vi "unset seq channel writer or reader.vi"(7 "action GUID":string, 8 "error in":errorcluster, 9 "action channel":refnum<class "TBM channel.lvclass">, 10 "seq channel":refnum<class "TBM channel.lvclass">, 11 "engine configuration in":refnum<class "base TBM sequencer configuration.lvclass">) -> (0 "error out":errorcluster, 3 "engine configuration out":refnum<class "base TBM sequencer configuration.lvclass">)   [LabVIEW 2014, in "base TBM sequencer configuration.lvclass"]
uses:
  base TBM sequencer configuration.lvclass
  <vilib>/NI/Tag Bus Module Framework/channel/TBM channel.lvclass
  <vilib>/NI/Tag Bus/tag/tag descriptor.lvclass/tag descriptor.ctl
  base TBM sequencer configuration.lvclass/base TBM sequencer configuration.ctl
  <vilib>/NI/Tag Bus Module Framework/channel/TBM channel.lvclass/TBM channel.ctl
  <vilib>/NI/Tag Bus/tag/read tag name.vi
  <vilib>/NI/Tag Bus Module Framework/channel/Read channel classification.vi
  <vilib>/NI/Configuration Framework/NISE_CEF_TreeControl.lvlib
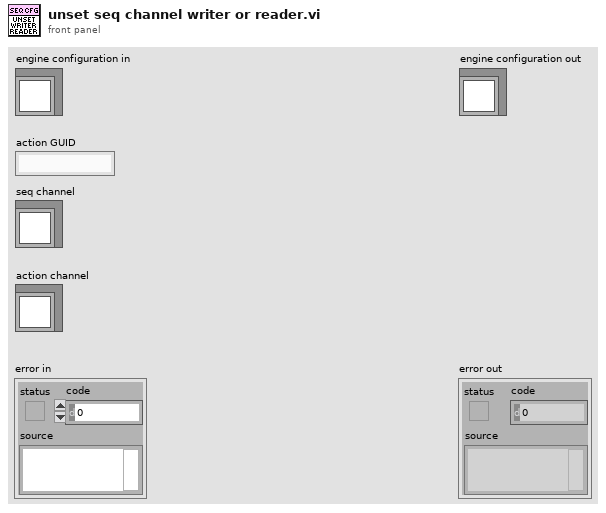
[diagram p1: front panel]
types:
  T1 = typedef "base TBM sequencer configuration.lvclass/Tag Info.ctl" = cluster{"Channel":refnum<class "TBM channel.lvclass">, "Writers":string[], "Readers":string[], "Owning ID":string}
  T2 = typedef "TBM channel.lvclass/channel classification.ctl" = enum16{"input data", "output data", "processing parameter", "processing result"}
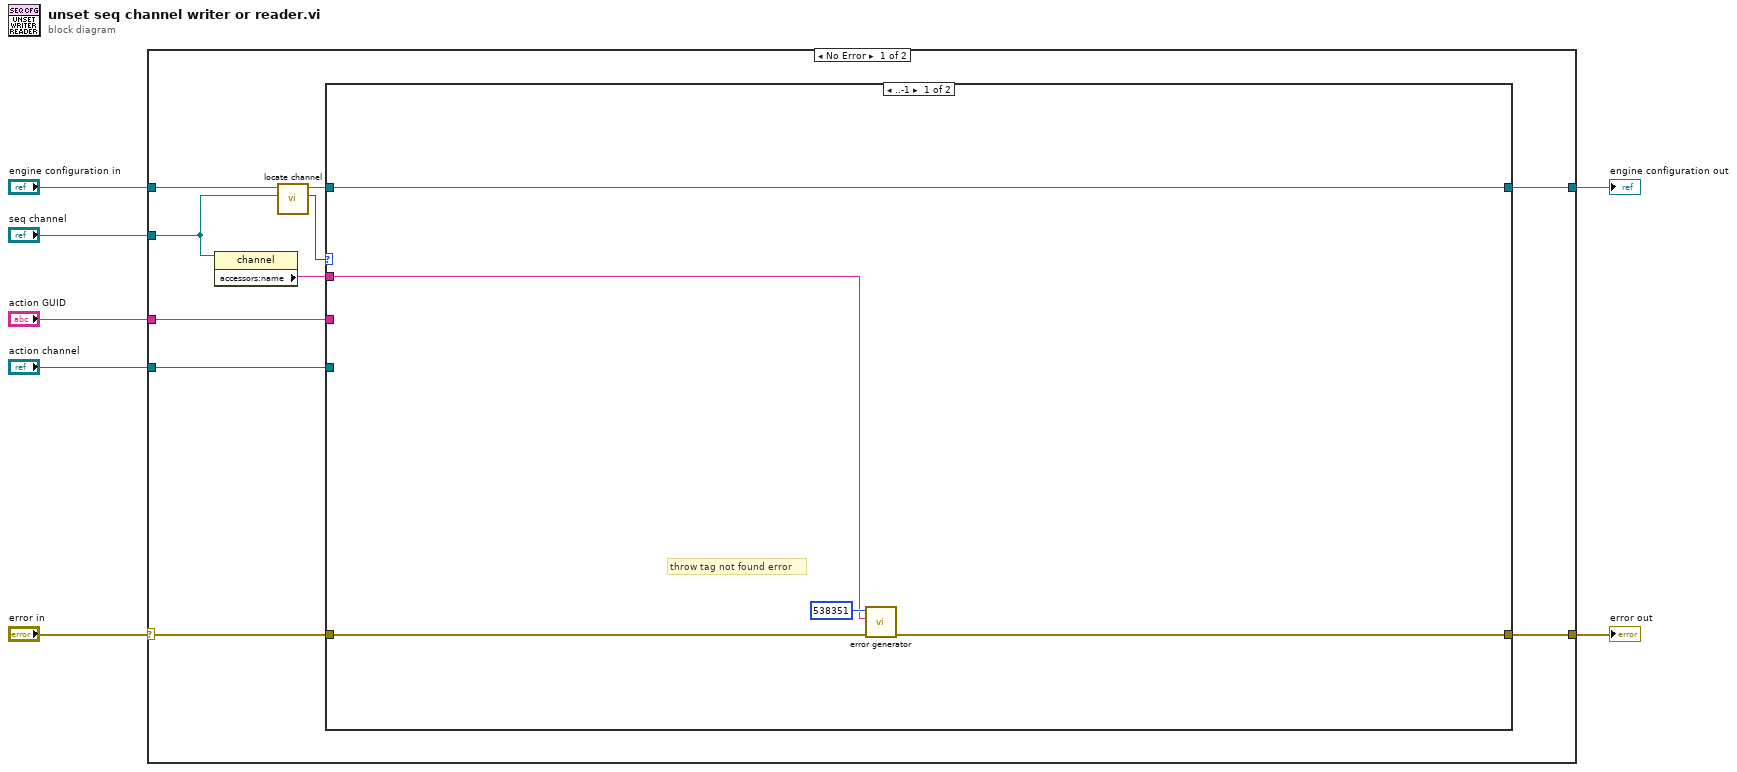
[diagram p0: block diagram]
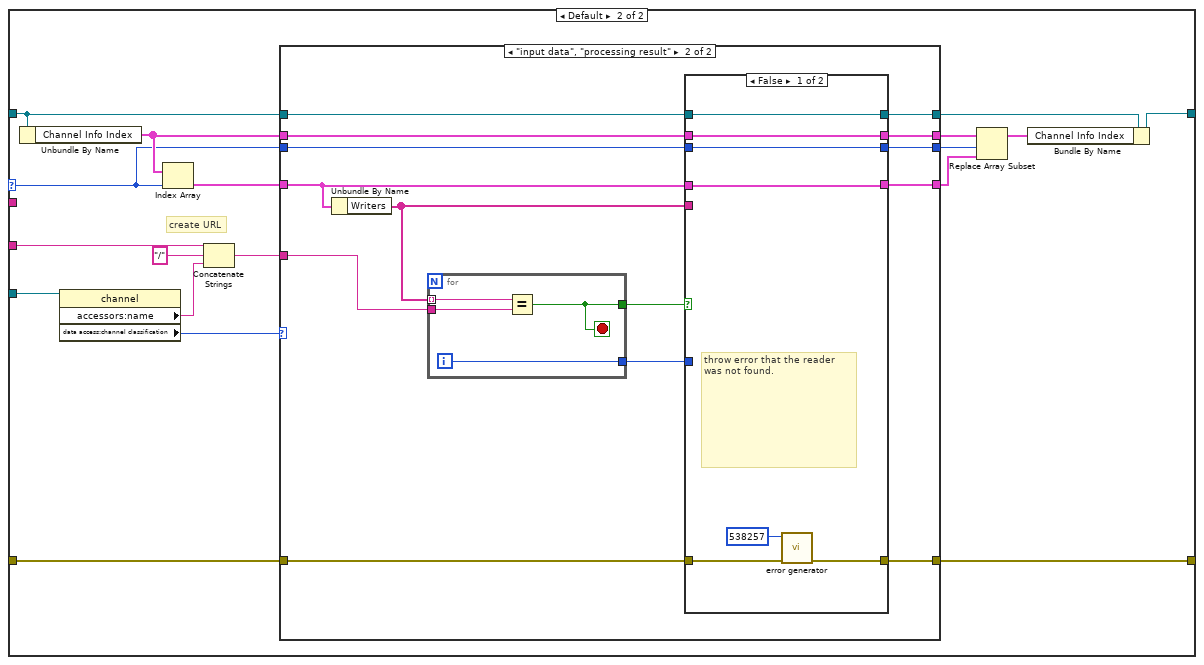
[diagram p2: hidden frame]
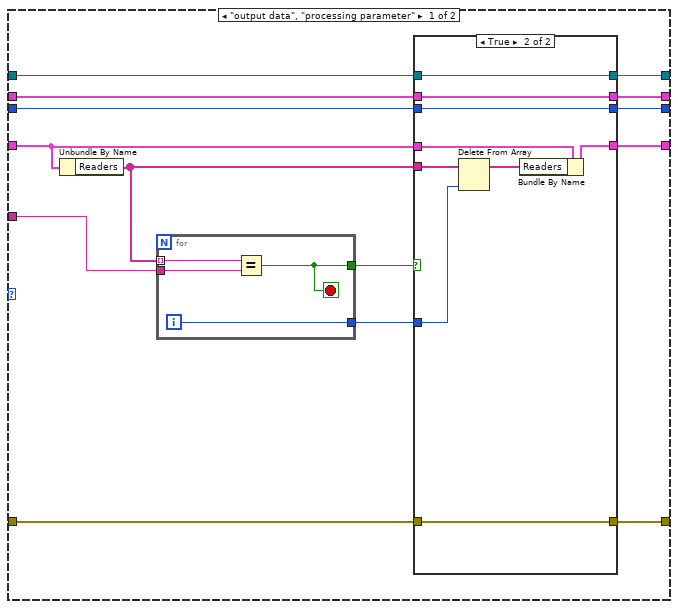
[diagram p3: hidden frame]
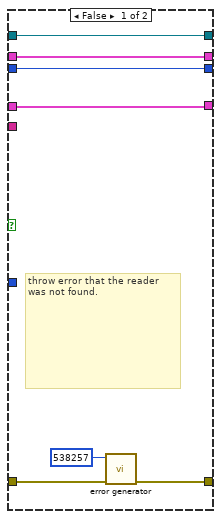
[diagram p4: hidden frame]
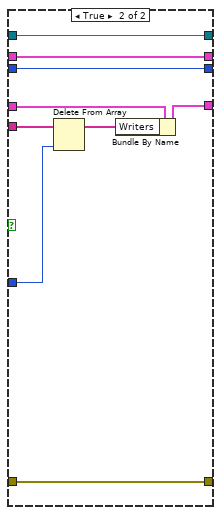
[diagram p5: hidden frame]
diagram:
  n1 = case shown="No Error" "error in" {
    selector: "error in" -> [w13 w110]
    tunnel: [w11 w110] -> w6
    tunnel: [w10 w109] -> w4
    tunnel: "engine configuration in" -> [w17 w109]
    tunnel: "seq channel" -> [w9 _]
    tunnel: "action GUID" -> [w14 _]
    tunnel: "action channel" -> [w15 _]
    frame No Error {
      n2 = property class="channel"(reference=w9) -> ("accessors:name"=w8:string)  [unwired: 1 in, 2 out]
      n3 = call "locate channel.vi"("tag descriptor"=w9, "sequencer config in"=w17) -> ("index"=w12:i32, "sequencer config out"=w16:refnum<class "base TBM sequencer configuration.lvclass">)  [unwired: 8 in]
      n4 = case shown="..-1" w12 {
        selector: w12 -> [_ w31]
        tunnel: w16 -> [w22 w30]
        tunnel: w15 -> [_ w40]
        tunnel: w14 -> [_ w38]
        tunnel: w13 -> [w20 w33]
        tunnel: [w19 w29] -> w11
        tunnel: [w22 w23] -> w10
        tunnel: w8 -> [w18 _]
        frame ..-1 {
          # "throw tag not found error"
          n5 = call <vilib>:"error generator.vi"("error in"=w20, "append error message"=w18, "error code (0)"=538351) -> ("error out"=w19:errorcluster)  [unwired: 6 in]
        }
        frame Default {
          # "create URL"
          n6 = Unbundle By Name(w30) -> ("Channel Info Index"=w32:T1[])
          n7 = property class="channel"(reference=w40) -> ("accessors:name"=w37:string, "data access:channel classification"=w36:T2)  [unwired: 1 in, 2 out]
          n8 = Index Array(array=w32, index=w31) -> (element=w34:T1)
          n9 = Concatenate Strings(w38, "/" ("string"), w37) -> (w35:string)
          n10 = case shown="\"input data\", \"processing result\"" w36 {
            tunnel: w35 -> [w52 w86]
            tunnel: w34 -> [w51 w85]
            tunnel: w33 -> [w47 w81]
            tunnel: w32 -> [w44 w78]
            tunnel: w31 -> [w42 w76]
            tunnel: w30 -> [w50 w84]
            tunnel: [w49 w83] -> w25
            tunnel: [w48 w82] -> w26
            tunnel: [w46 w80] -> w29
            tunnel: [w45 w79] -> w27
            tunnel: [w43 w77] -> w28
            frame "output data", "processing parameter" {
              n11 = Unbundle By Name(w51) -> ("Readers"=w53:string[])
              n12 = for {
                tunnel: w53 -> [w73] mode=indexing
                tunnel: w52 -> [w74]
                tunnel: [w72] -> w54
                tunnel: [w71] -> w41
                i -> [w71]
                stop <- w72 stop-if-true
                n13 = Equal?(x=w73, y=w74) -> (x = y?=w72:bool)
              }
              n14 = case shown="True" w54 {
                tunnel: w53 -> [_ w64]
                tunnel: w51 -> [w60 w70]
                tunnel: w50 -> [w61 w69]
                tunnel: [w61 w69] -> w49
                tunnel: [w60 w68] -> w48
                tunnel: w47 -> [w56 w67]
                tunnel: [w55 w67] -> w46
                tunnel: [w59 w66] -> w45
                tunnel: w44 -> [w59 w66]
                tunnel: [w58 w65] -> w43
                tunnel: w42 -> [w58 w65]
                tunnel: w41 -> [_ w62]
                frame False {
                  # "throw error that the reader was not found."
                  n15 = call <vilib>:"error generator.vi"("error in"=w56, "error code (0)"=538257) -> ("error out"=w55:errorcluster)  [unwired: 7 in]
                }
                frame True {
                  n16 = Delete From Array(array=w64, index=w62) -> (array with subset deleted=w63:string[])  [unwired: 1 in, 1 out]
                  n17 = Bundle By Name(cluster=w70, "Readers"=w63) -> (w68:T1)
                }
              }
            }
            frame "input data", "processing result" {
              n18 = Unbundle By Name(w85) -> ("Writers"=w87:string[])
              n19 = for {
                tunnel: w87 -> [w107] mode=indexing
                tunnel: w86 -> [w108]
                tunnel: [w106] -> w88
                tunnel: [w105] -> w75
                i -> [w105]
                stop <- w106 stop-if-true
                n20 = Equal?(x=w107, y=w108) -> (x = y?=w106:bool)
              }
              n21 = case shown="False" w88 {
                tunnel: w87 -> [_ w98]
                tunnel: w85 -> [w94 w104]
                tunnel: w84 -> [w95 w103]
                tunnel: [w95 w103] -> w83
                tunnel: [w94 w102] -> w82
                tunnel: w81 -> [w90 w101]
                tunnel: [w89 w101] -> w80
                tunnel: [w93 w100] -> w79
                tunnel: w78 -> [w93 w100]
                tunnel: [w92 w99] -> w77
                tunnel: w76 -> [w92 w99]
                tunnel: w75 -> [_ w96]
                frame False {
                  # "throw error that the reader was not found."
                  n22 = call <vilib>:"error generator.vi"("error in"=w90, "error code (0)"=538257) -> ("error out"=w89:errorcluster)  [unwired: 7 in]
                }
                frame True {
                  n23 = Delete From Array(array=w98, index=w96) -> (array with subset deleted=w97:string[])  [unwired: 1 in, 1 out]
                  n24 = Bundle By Name(cluster=w104, "Writers"=w97) -> (w102:T1)
                }
              }
            }
          }
          n25 = Replace Array Subset(array=w27, new element=w26, index=w28) -> (w24:T1[])
          n26 = Bundle By Name(cluster=w25, "Channel Info Index"=w24) -> (w23:refnum<class "base TBM sequencer configuration.lvclass">)
        }
      }
    }
    frame Error {
    }
  }
  "error out" <- w6
  "engine configuration out" <- w4
